vi "Write BIO.vi"(8 "error in (no error)":errorcluster, 10 "SSL_Lib.lvlib:BIO.lvclass":refnum<class "BIO.lvclass">, 11 "SSL Socket in":refnum<class "SSL Socket.lvclass">) -> (0 "error out":errorcluster, 3 "SSL Socket out":refnum<class "SSL Socket.lvclass">)   [LabVIEW 2013, in "OpenSSL Socket.lvlib" / "SSL Socket.lvclass"]
uses:
  SSL Socket.lvclass
  SSL_Lib/BIO/BIO.lvclass
  SSL Socket.lvclass/SSL Socket.ctl
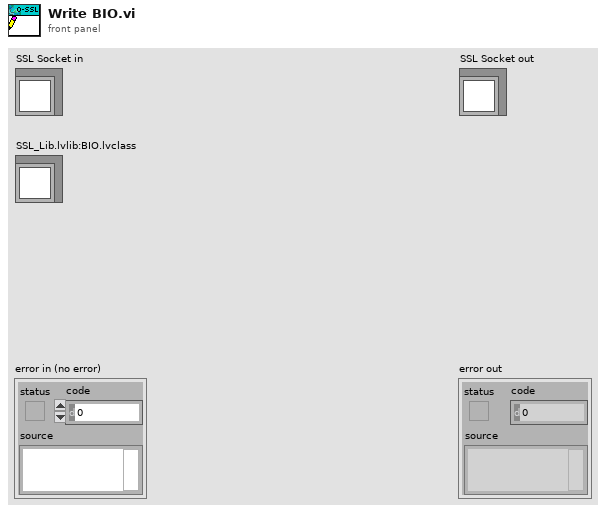
[diagram p1: front panel]
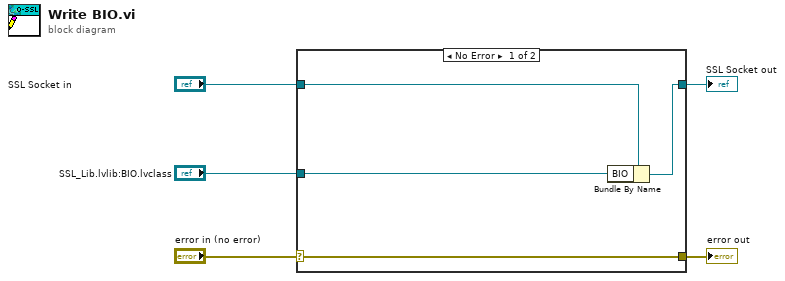
[diagram p0: block diagram]
diagram:
  n1 = case shown="No Error" "error in (no error)" {
    selector: "error in (no error)" -> [w9 w10]
    tunnel: [w9 w10] -> w4
    tunnel: [w7 w11] -> w2
    tunnel: "SSL Socket in" -> [w8 w11]
    tunnel: "SSL_Lib.lvlib:BIO.lvclass" -> [w6 _]
    frame No Error {
      n2 = Bundle By Name(cluster=w8, "BIO"=w6) -> (w7:refnum<class "SSL Socket.lvclass">)
    }
    frame Error {
    }
  }
  "error out" <- w4
  "SSL Socket out" <- w2
